vi "Write CmdLib.vi"(8 "error in (no error)":errorcluster, 10 "CmdLib":refnum<k24>, 11 "2936r in":refnum<class "2936r.lvclass">) -> (0 "error out":errorcluster, 3 "2936r out":refnum<class "2936r.lvclass">)   [LabVIEW 2018, in "2936r.lvlib" / "2936r.lvclass"]
uses:
  2936r.lvclass
  C:/Projects/LabVIEW/Built/Optical Power Meter/2936R/Required library/PowerMeterCommands.dll
  Required library/PowerMeterCommands.dll
  2936r.lvclass/2936r.ctl
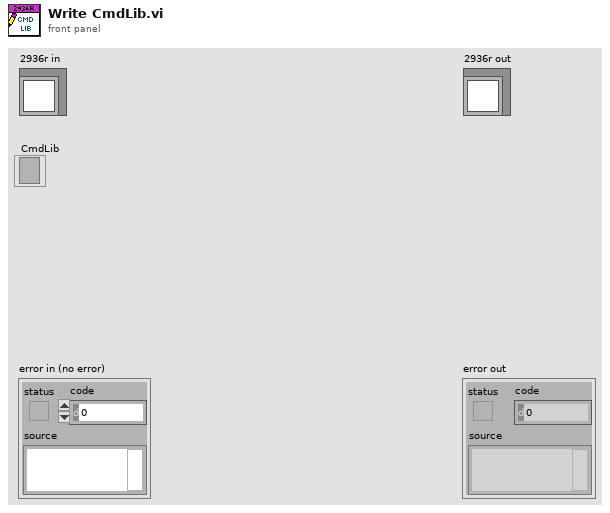
[diagram p1: front panel]
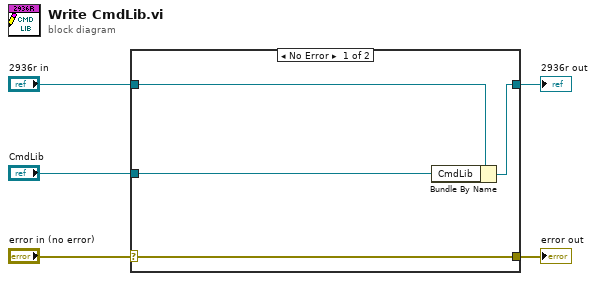
[diagram p0: block diagram]
diagram:
  n1 = case shown="No Error" "error in (no error)" {
    selector: "error in (no error)" -> [w9 w10]
    tunnel: [w9 w10] -> w4
    tunnel: [w7 w11] -> w2
    tunnel: "2936r in" -> [w8 w11]
    tunnel: "CmdLib" -> [w6 _]
    frame No Error {
      n2 = Bundle By Name(cluster=w8, "CmdLib"=w6) -> (w7:refnum<class "2936r.lvclass">)
    }
    frame Error {
    }
  }
  "error out" <- w4
  "2936r out" <- w2
